vi "Launch Actor.vi"(4 "Debug Alias":string, 6 "Open Actor Core front panel? (F)":bool, 8 "error in (no error)":errorcluster, 10 "Actor-to-Caller Enqueuer":refnum<class "Message Enqueuer.lvclass">, 11 "Actor":refnum<class "Actor.lvclass">) -> (0 "error out":errorcluster, 3 "Caller-To-Actor Enqueuer":refnum<class "Message Enqueuer.lvclass">)   [LabVIEW 2020, in "Actor Framework.lvlib" / "Actor.lvclass"]
doc: "LabVIEW no longer supports this VI. Use the Actor:Launch Root Actor VI or Actor:Launch Nested Actor VI instead.\nLaunches a top-level VI that handles messages for an actor and starts this actor's tasks. This VI returns a reference to the queue you use to send messages to the actor.\n\nThis VI requires the <B>Actor-to-Caller Enqueuer</B> input, which is the reference that allows the launched actor to communicate with the caller. If you are launching the top-level actor, use the Read Enqueuer method to obtain this reference. If you are launching a nested actor, use the Read Self Enqueuer method instead."
uses:
  <vilib>/ActorFramework/Actor/Actor.lvclass
  <vilib>/ActorFramework/Message Enqueuer/Message Enqueuer.lvclass
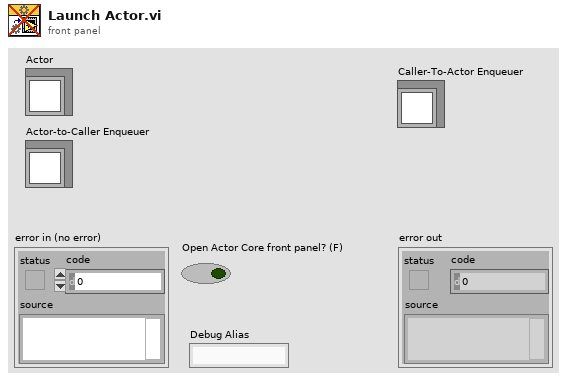
[diagram p1: front panel]
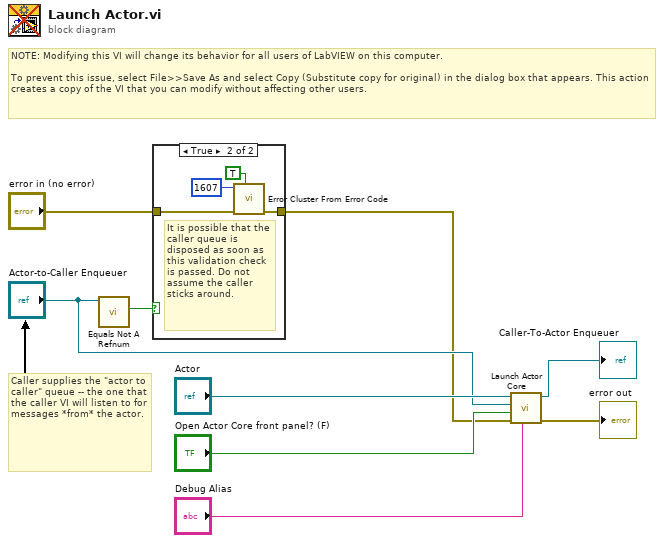
[diagram p0: block diagram]
diagram:
  # "Caller supplies the \"actor to caller\" queue -- the one that the caller VI will listen to for messages *from* the actor."
  # "NOTE: Modifying this VI will change its behavior for all users of LabVIEW on this computer.\n\nTo prevent this issue, select File>>Save As and select Copy (Substitute copy for original) in the dialog box that appears. This action creates a copy of the VI that you can modify without affecting other users."
  n1 = call <vilib>:"Equals Not A Refnum.vi"("Message Enqueuer"="Actor-to-Caller Enqueuer") -> ("Not a refnum?"=w8:bool)  [unwired: 10 in]
  n2 = case shown="True" w8 {
    tunnel: "error in (no error)" -> [w10 w14]
    tunnel: [w10 w13] -> w4
    frame False {
    }
    frame True {
      # "It is possible that the caller queue is disposed as soon as this validation check is passed. Do not assume the caller sticks around."
      n3 = call <vilib>:"Error Cluster From Error Code.vi"("show call chain? (False)"=TRUE, "error in (no error)"=w14, "error code (0)"=1607) -> ("error out"=w13:errorcluster)  [unwired: 6 in]
    }
  }
  n4 = call <vilib>:"Launch Actor Core.vi"("Debug Alias"="Debug Alias", "error in (no error)"=w4, "Open Actor Core front panel?"="Open Actor Core front panel? (F)", "Caller's Enqueuer"="Actor-to-Caller Enqueuer", "Actor in"="Actor") -> ("error out"=→"error out":errorcluster, "Message Enqueuer out"=→"Caller-To-Actor Enqueuer":refnum<class "Message Enqueuer.lvclass">)  [unwired: 5 in]
